vi "TCP_Close.vi"(8 "error in (no error) 2":errorcluster) -> (0 "error out":errorcluster)   [LabVIEW 2022 SP3]
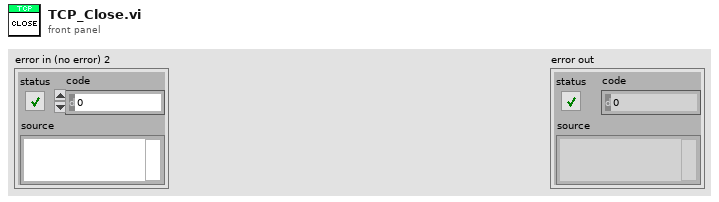
[diagram p1: front panel]
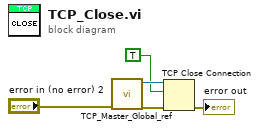
[diagram p0: block diagram]
diagram:
  n1 = call "TCP_Master_Global_ref.vi"("error in (no error) 2"="error in (no error) 2") -> ("error out 2"=w4:errorcluster, "ID OUT"=w5:refnum<k5>)  [unwired: 9 in]
  n2 = TCP Close Connection(connection ID=w5, abort (F)=TRUE, error in (no error)=w4) -> (error out=→"error out":errorcluster)  [unwired: 1 out]
